vi "TestSSM.vi"() -> ()   [LabVIEW 2018, in "Test.lvclass"]
uses:
  Test.lvclass
  Test.lvclass/Test.ctl
  Accessors/Write ModuleIDs.vi
panel:
  out "found?":bool
  out "error out":errorcluster
  in  "ModuleList":string[](array[string])=["AcPwr.Chroma"]
  in  "ModuleIDs":i32[](array[numeric])=[4140002]
  in  "Tab Control":enum32{"CommandsFromFile", "Manual Entry"}(tab)
  in  "File Path Control":path=path "C:/Users/ico/Downloads/Test.txt"
  in  "Commands":string[](array[string])
  in  "Commands To Loop":string[](array[string])=["AcPwrDeviceOn,Chroma", "Delay,2000", "AcPwrDeviceOff,Chroma", "Delay,2000"]
  in  "NumberOfLoops":i32=2
  in  "Loop Commands Insertion Index":i32=5
  out "Commands Sent To SSM":string[](array[string])=["AcPwrInit", "AcPwrConfig", "AcPwrStartMeas,PPS,1", "AcPwrStartMeas,Chroma", "AcPwrDeviceOn,Chroma", "Delay,2000", "AcPwrDeviceOff,Chroma", "Delay,2000", "AcPwrDeviceOn,Chroma", "Delay,2000", "AcPwrDeviceOff,Chroma", "Delay,2000", "AcPwrDeviceOn,PPS", "AcPwrDeviceOff,PPS", "AcPwrClose,PPS", "AcPwrClose,Chroma", "Stop"]
  in  "Running?":bool
  out "Data":variant=variant(string[] [])
  out "ErrorArray":errorcluster[](array[cluster])
  # "True if a Framework is controlling the modules. False if uisng the TestCloneAPI to make the modules"
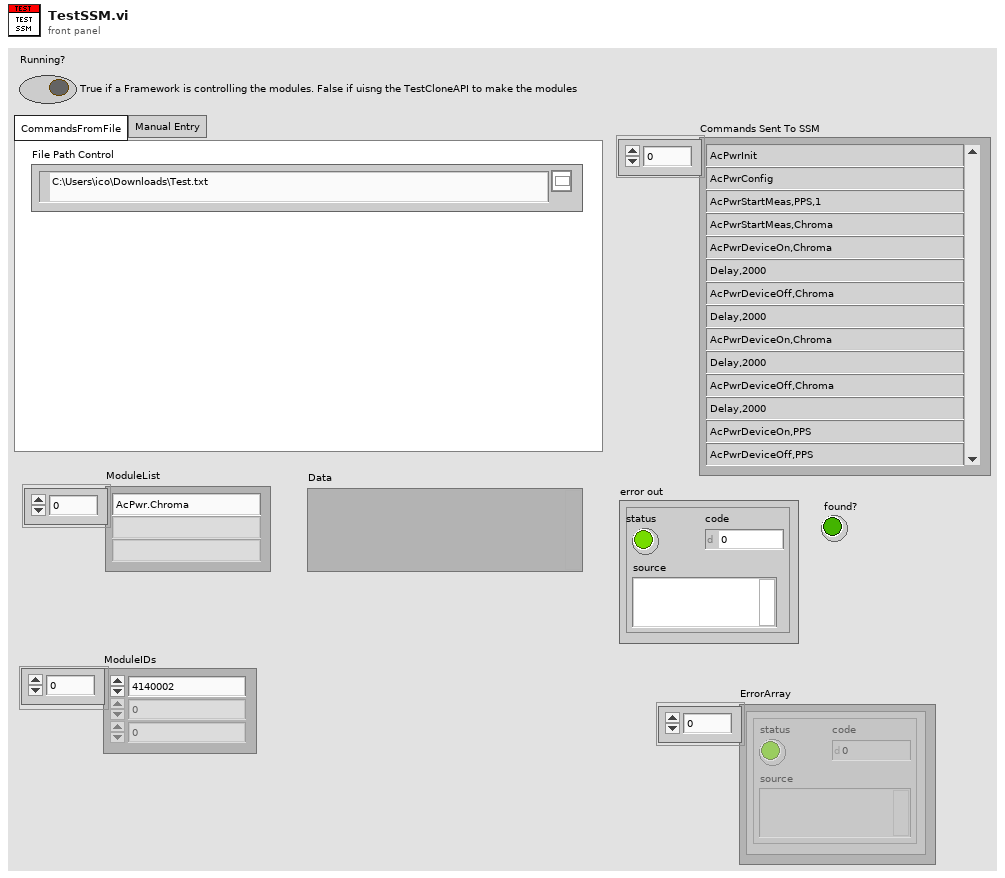
[diagram p1: front panel]
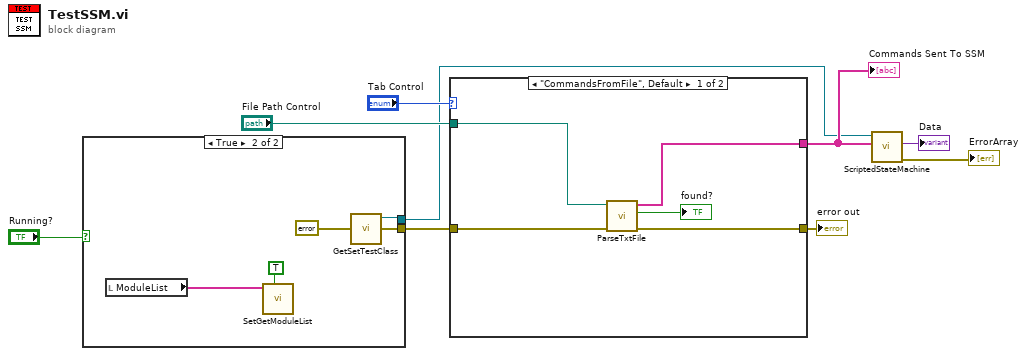
[diagram p0: block diagram]
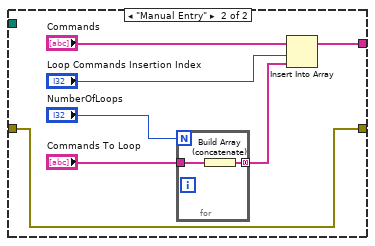
[diagram p2: hidden frame]
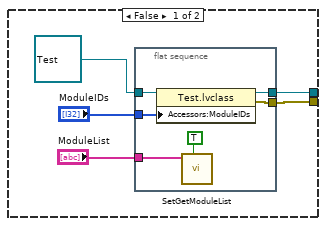
[diagram p3: hidden frame]
diagram:
  n1 = case shown="True" "Running?" {
    tunnel: [w12 w24] -> w2
    tunnel: [w10 errorcluster {"status"=FALSE, "code"=0, "source"=""} ("error out")] -> w3
    frame False {
      n2 = flat-sequence {
        tunnel: refnum<class "Test.lvclass"> refnum ("Test.lvclass") -> [w20]
        tunnel: "ModuleIDs" -> [w19]
        tunnel: [w18] -> w12
        tunnel: "ModuleList" -> [w17]
        tunnel: [w15] -> w10
        frame #0 {
          n3 = property class="Test.lvclass"(reference=w20, "Accessors:ModuleIDs"=w19) -> (reference out=w18:refnum<class "Test.lvclass">, error out=w15:errorcluster)  [unwired: 1 in]
          n4 = call "SetGetModuleList.vi"("Set? (F)"=TRUE ("Set? (f)"), "ModuleList"=w17) -> ()  [unwired: 9 in, 1 out]
        }
      }
    }
    frame True {
      n5 = local read "ModuleList"() -> (w21:string[])
      n6 = call "SetGetModuleList.vi"("Set? (F)"=TRUE ("Set? (f)"), "ModuleList"=w21) -> ()  [unwired: 9 in, 1 out]
      n7 = call "GetSetTestClass.vi"() -> ("Test.lvclass"=w24:refnum<class "Test.lvclass">)  [unwired: 11 in]
    }
  }
  n8 = case shown="\"CommandsFromFile\", Default" "Tab Control" {
    tunnel: [w26 w33] -> w6
    tunnel: "File Path Control" -> [w29 _]
    tunnel: w3 -> [w28 w30]
    tunnel: [w27 w30] -> w1
    frame "CommandsFromFile", Default {
      n9 = call "ParseTxtFile.vi"("error in"=w28, "file path (use dialog)"=w29) -> ("error out"=w27:errorcluster, "found?"=→"found?":bool, "Commands Sent To SSM"=w26:string[])  [unwired: 7 in]
    }
    frame "Manual Entry" {
      n10 = for {
        N: "NumberOfLoops" -> [_]
        tunnel: "Commands To Loop" -> [w38]
        tunnel: [w37] -> w31 mode=concatenating
        n11 = Build Array (concatenate)(w38) -> (w37:string[])
      }
      n12 = Insert Into Array(array="Commands", index="Loop Commands Insertion Index", new element=w31) -> (w33:string[])
    }
  }
  "Commands Sent To SSM" <- w6
  "error out" <- w1
  n13 = call "ScriptedStateMachine.vi"("script"=w6, "Test.lvclass"=w2) -> ("ErrorArray"=→"ErrorArray":errorcluster[], "Data"=→"Data":variant)  [unwired: 7 in, 1 out]
